vi "拖拽控件.vi"(8 "error in (no error)":errorcluster caption="错误输入（无错误）", 11 "程序响应 输入":refnum<class "程序响应.lvclass">) -> (0 "error out":errorcluster caption="错误输出", 3 "程序响应 输出":refnum<class "程序响应.lvclass">)   [LabVIEW 2020, in "程序响应.lvlib" / "程序响应.lvclass"]
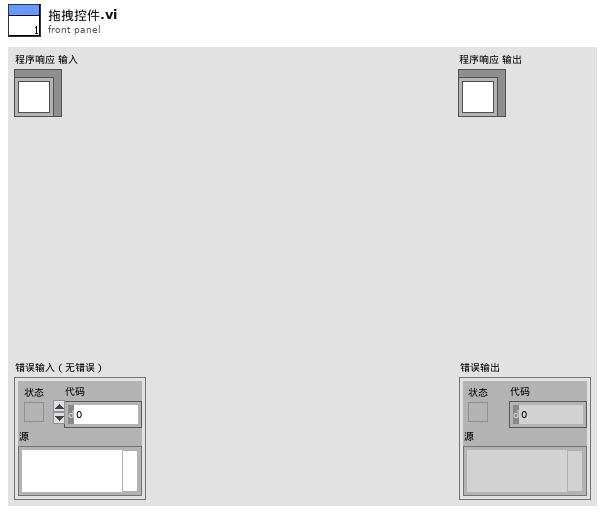
[diagram p1: front panel]
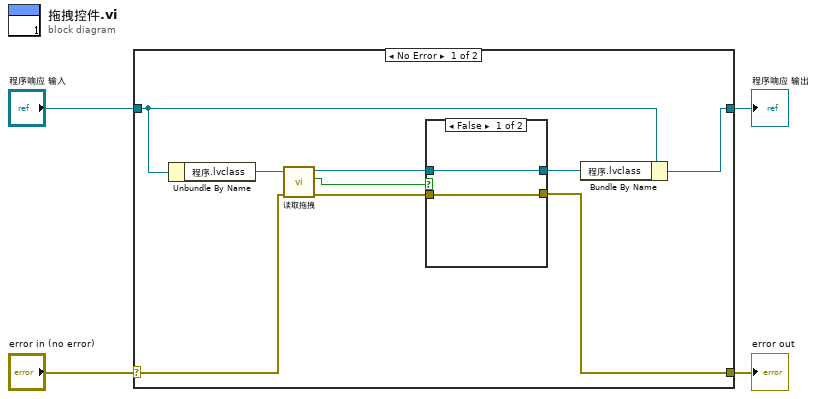
[diagram p0: block diagram]
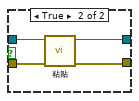
[diagram p2: hidden frame]
diagram:
  n1 = case shown="No Error" "error in (no error)" {
    selector: "error in (no error)" -> [w9 w21]
    tunnel: [w6 w21] -> w3
    tunnel: [w5 w20] -> w1
    tunnel: "程序响应 输入" -> [w8 w20]
    frame No Error {
      n2 = Unbundle By Name(w8) -> ("程序.lvclass"=w13:refnum<class "程序.lvclass">)
      n3 = call-dynamic "读取拖拽.vi"("error in (no error)"=w9, "程序输入"=w13) -> ("error out"=w10:errorcluster, "拖拽"=w12:bool, "程序输出"=w11:refnum<class "程序.lvclass">)  [unwired: 7 in]
      n4 = case shown="False" w12 {
        tunnel: w11 -> [w15 w19]
        tunnel: w10 -> [w14 w18]
        tunnel: [w15 w17] -> w7
        tunnel: [w14 w16] -> w6
        frame False {
        }
        frame True {
          n5 = call-dynamic "粘贴.vi"("error in (no error)"=w18, "程序 输入"=w19) -> ("error out"=w16:errorcluster, "程序 输出"=w17:refnum<class "程序.lvclass">)  [unwired: 8 in]
        }
      }
      n6 = Bundle By Name(cluster=w8, "程序.lvclass"=w7) -> (w5:refnum<class "程序响应.lvclass">)
    }
    frame Error {
    }
  }
  "error out" <- w3
  "程序响应 输出" <- w1
